vi "sub_intitializePuzzleSolverArray.vi"(8 "error in (no error)":errorcluster, 10 "solver array":cluster{"solved":bool, "values":string[]}[][](array[cluster]), 11 "puzzle (in)":string[][](array[string])) -> (0 "error out":errorcluster, 2 "solver array 2":cluster{"solved":bool, "values":string[]}[][](array[cluster]))   [LabVIEW 2018]
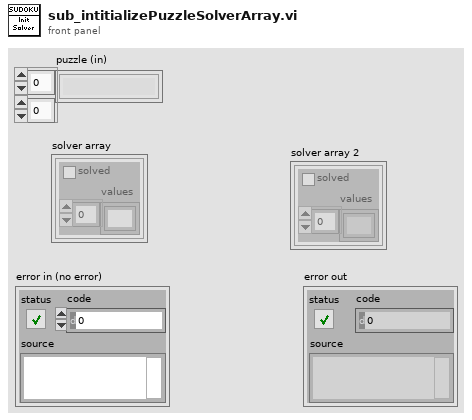
[diagram p1: front panel]
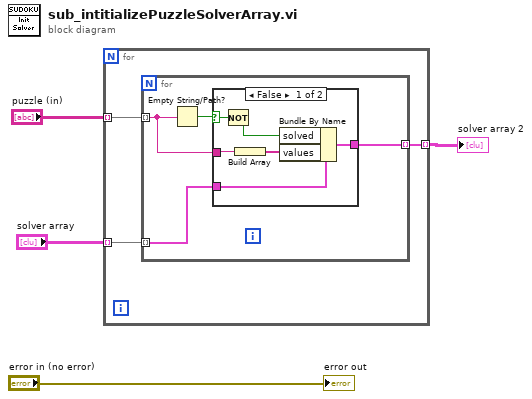
[diagram p0: block diagram]
diagram:
  n1 = for {
    tunnel: "puzzle (in)" -> [w7] mode=indexing
    tunnel: "solver array" -> [w6] mode=indexing
    tunnel: [w5] -> w2 mode=indexing
    n2 = for {
      tunnel: w7 -> [w9] mode=indexing
      tunnel: w6 -> [w10] mode=indexing
      tunnel: [w8] -> w5 mode=indexing
      n3 = Empty String/Path?(string/path=w9) -> (empty?=w11:bool)
      n4 = case shown="False" w11 {
        selector: w11 -> [w16 _]
        tunnel: w10 -> [w17 w18]
        tunnel: w9 -> [w14 _]
        tunnel: [w12 w18] -> w8
        frame False {
          n5 = Not(x=w16) -> (.not. x?=w15:bool)
          n6 = Build Array(w14) -> (w13:string[])
          n7 = Bundle By Name(cluster=w17, "solved"=w15, "values"=w13) -> (w12:cluster{"solved":bool, "values":string[]})
        }
        frame True {
        }
      }
    }
  }
  "solver array 2" <- w2
  "error out" <- "error in (no error)"
